vi "init daq state.vi"(7 "DAQ state start in":T6 {"T cont"."utility"."therm volt" format="%_6g"; "T cont"."utility"."heat volt in" format="%_6g"; "T cont"."utility"."heat volt out" format="%_6g"; "T cont"."utility"."power out" format="%_6g"; "T cont"."utility"."H Vmax" format="%_6g"; "T cont"."exec"."man power" format="%_6g"; "T cont"."T status"."Power" format="%_6g"; "T cont"."T status"."Temp" format="%_6g"}, 11 "T cont wait time (ms)":i32=300) -> (4 "T cont out for global update":T1={"exec"={"T mode"=enum."Listening to exec", "man power"=0.5, "log"=FALSE}, "T status"={"Temp"=0.0, "Power"=0.0}, "utility"={"meas index"=0, "wait (ms)"=300, "H Vmax"=8.5, "power out"=0.0, "heat volt out"=0.0, "heat volt in"=0.0, "therm volt"=0.0, "t T P hist"=[]}} {"utility"."therm volt" format="%_6g"; "utility"."heat volt in" format="%_6g"; "utility"."heat volt out" format="%_6g"; "utility"."power out" format="%_6g"; "utility"."H Vmax" format="%_6g"; "exec"."man power" format="%_6g"; "T status"."Power" format="%_6g"; "T status"."Temp" format="%_6g"}, 8 "DAQ state start out":T6 {"T cont"."utility"."therm volt" format="%_6g"; "T cont"."utility"."heat volt in" format="%_6g"; "T cont"."utility"."heat volt out" format="%_6g"; "T cont"."utility"."power out" format="%_6g"; "T cont"."utility"."H Vmax" format="%_6g"; "T cont"."exec"."man power" format="%_6g"; "T cont"."T status"."Power" format="%_6g"; "T cont"."T status"."Temp" format="%_6g"})   [LabVIEW 2019]
doc: "Thus subvi initializes the temp daq state machine and the global variables for the bug experiment.\n\nPaul K Dixon\nP3600\nCSUSB Physics"
uses:
  typedefs/DAQ T state cluster.ctl
  typedefs/DAQ T state enum.ctl
  typedefs/temp cont cluster.ctl
  typedefs/temp exec cluster.ctl
  typedefs/temp mode enum.ctl
  typedefs/temp indicator.ctl
  typedefs/temp cont utility.ctl
panel:
  in  "T cont.T status":T4={"Temp"=25.0, "Power"=0.0} {"Power" format="%_6g"; "Temp" format="%_6g"}
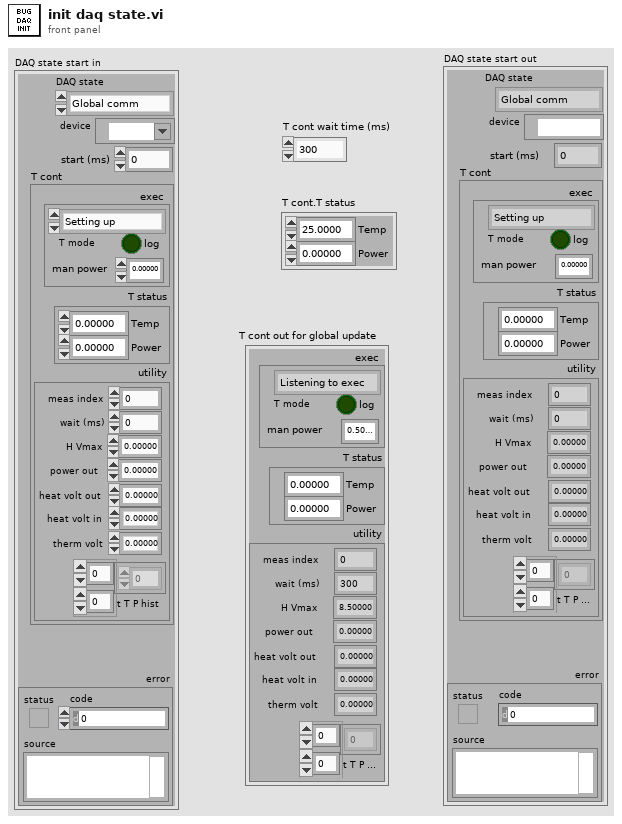
[diagram p1: front panel]
types:
  T1 = typedef "temp cont cluster.ctl" = cluster{"exec":T2, "T status":T4, "utility":T5}
  T2 = typedef "temp exec cluster.ctl" = cluster{"T mode":T3, "man power":dbl, "log":bool}
  T3 = typedef "temp mode enum.ctl" = enum16{"Setting up", "Listening to exec", "Exit"}
  T4 = typedef "temp indicator.ctl" = cluster{"Temp":dbl, "Power":dbl}
  T5 = typedef "temp cont utility.ctl" = cluster{"meas index":i32, "wait (ms)":i32, "H Vmax":dbl, "power out":dbl, "heat volt out":dbl, "heat volt in":dbl, "therm volt":dbl, "t T P hist":dbl[][]}
  T6 = typedef "DAQ T state cluster.ctl" = cluster{"DAQ state":T7, "device":tag, "start (ms)":i32, "error":errorcluster, "T cont":T1}
  T7 = typedef "DAQ T state enum.ctl" = enum16{"Global comm", "Meas T & P", "Man Power set", "Output Power", "Wait", "Exit"}
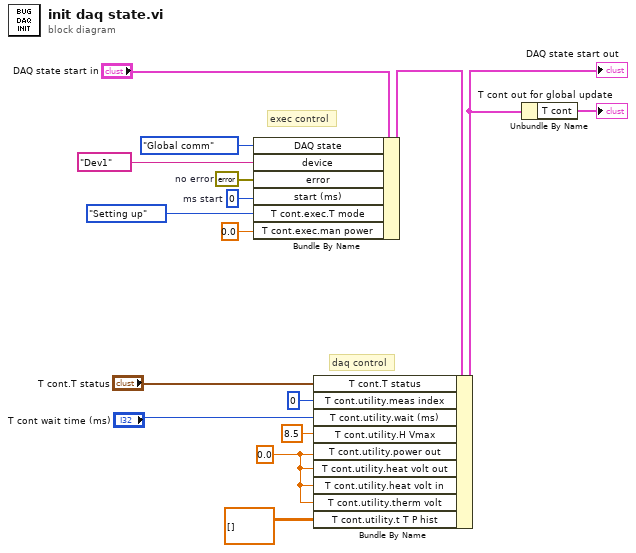
[diagram p0: block diagram]
diagram:
  w4 = 0.0 ("T cont.H Vmax")
  w10 = u32 0  # ms start
  w13 = errorcluster {"status"=FALSE, "code"=0, "source"=""}  # no error
  # "daq control"
  # "exec control"
  n1 = Bundle By Name(cluster="DAQ state start in", "DAQ state"=DAQ_T_state_enum."Global comm", "device"=tag "Dev1", "error"=w13, "start (ms)"=w10, "T cont.exec.T mode"=temp_mode_enum."Setting up", "T cont.exec.man power"=0.0) -> (w12:T6)
  n2 = Bundle By Name(cluster=w12, "T cont.T status"="T cont.T status", "T cont.utility.meas index"=0 ("T cont.therm volt"), "T cont.utility.wait (ms)"="T cont wait time (ms)", "T cont.utility.H Vmax"=8.5 ("T cont.H Vmax"), "T cont.utility.power out"=w4, "T cont.utility.heat volt out"=w4, "T cont.utility.heat volt in"=w4, "T cont.utility.therm volt"=w4, "T cont.utility.t T P hist"=dbl[][] [] ("T cont.T hist")) -> (w3:T6)
  "DAQ state start out" <- w3
  n3 = Unbundle By Name(w3) -> ("T cont"=→"T cont out for global update":T1)
